vi "Generate Text Icon.vi"(8 "error in (no error)":errorcluster, 11 "API VI Generator In":refnum<class "API VI Generator.lvclass">) -> (0 "error out":errorcluster, 3 "API VI Generator Out":refnum<class "API VI Generator.lvclass">)   [LabVIEW 2020, in "Method Generation.lvlib" / "API VI Generator.lvclass"]
uses:
  API VI Generator.lvclass
  API VI Generator.lvclass/API VI Generator.ctl
  Support/Support.lvlib
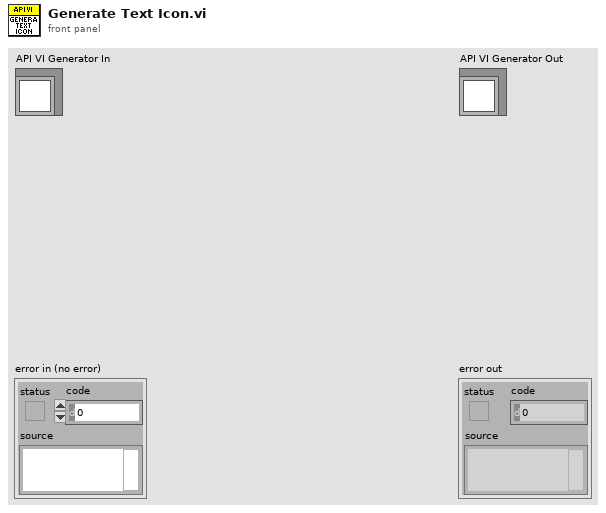
[diagram p1: front panel]
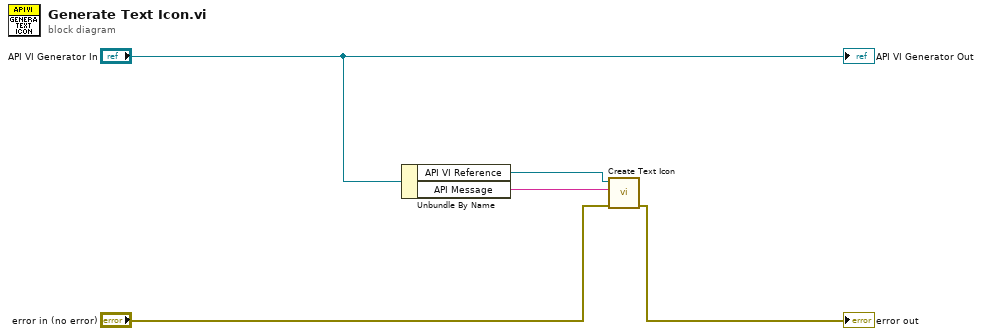
[diagram p0: block diagram]
diagram:
  n1 = Unbundle By Name("API VI Generator In") -> ("API VI Reference"=w4:refnum<vi>, "API Message"=w5:string)
  n2 = call "Create Text Icon.vi"("error in (no error)"="error in (no error)", "Icon Text String"=w5, "VI in"=w4) -> ("error out"=→"error out":errorcluster)  [unwired: 7 in, 1 out]
  "API VI Generator Out" <- "API VI Generator In"
